vi "OpenSERIAL.vi"(8 "error in (no error)":errorcluster, 9 "Update Rate (4Hz-100Hz)":u8=100, 10 "Protocol":T1=enum."AHRS", 11 "Serial Port":T2=enum."MXP TTL") -> (0 "error out":errorcluster, 3 "navX out":refnum<class "navX.lvclass">)   [LabVIEW 2015, in "navX Library v3.lvlib" / "navX.lvclass"]
uses:
  navX.lvclass
  _NI WPI Serial USB/WPI_SerialPort_USB.ctl
  navX - SERIAL/Protocol.ctl
  navX - SERIAL/navX - SERIAL.lvclass
  navX - SERIAL/navX - SERIAL.lvclass/navX - SERIAL.ctl
  navX - Interface/Notifications/Send Notification.vi
  _NI WPI Serial USB/_NI WPI Serial USB.lvlib
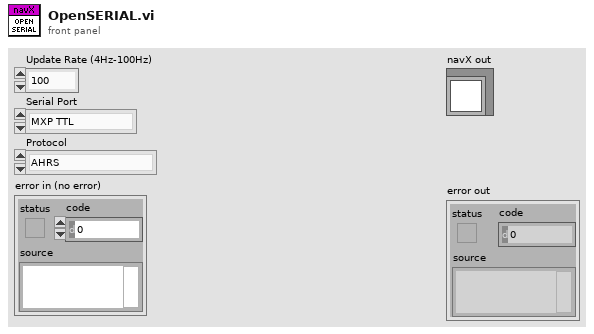
[diagram p1: front panel]
types:
  T1 = typedef "navX Library v3.lvlib/navX - SERIAL.lvclass/Protocol.ctl" = enum16{"YRPH", "Quaterinons", "Gyro/Raw", "AHRS", "AHRSAndPositioning"}
  T2 = typedef "_NI WPI Serial USB.lvlib/WPI_SerialPort_USB.ctl" = enum16{"Onboard RS-232", "MXP TTL", "USB"}
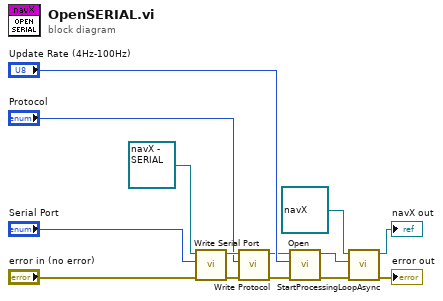
[diagram p0: block diagram]
diagram:
  n1 = call "Write Serial Port.vi"("error in (no error)"="error in (no error)", "Serial Port"="Serial Port", "navX - SERIAL in"=refnum<class "navX - SERIAL.lvclass"> refnum ("navX Library v3.lvlib:navX - SERIAL.lvclass")) -> ("error out"=w11:errorcluster, "navX - SERIAL out"=w12:refnum<class "navX - SERIAL.lvclass">)  [unwired: 7 in]
  n2 = call "Write Protocol.vi"("error in (no error)"=w11, "Protocol"="Protocol", "navX - SERIAL in"=w12) -> ("error out"=w8:errorcluster, "navX - SERIAL out"=w9:refnum<class "navX - SERIAL.lvclass">)  [unwired: 7 in]
  n3 = call-dynamic "Open.vi"("error in (no error)"=w8, "Update Rate (4Hz-100Hz)"="Update Rate (4Hz-100Hz)", "navX - SERIAL in"=w9) -> ("error out"=w5:errorcluster, "navX - SERIAL out"=w4:refnum<class "navX - SERIAL.lvclass">)  [unwired: 7 in]
  n4 = call "StartProcessingLoopAsync.vi"("error in (no error)"=w5, "navX Class in"=w4, "navX in"=refnum<class "navX.lvclass"> refnum ("navX Library v3.lvlib:navX.lvclass")) -> ("error out"=→"error out":errorcluster, "navX out"=→"navX out":refnum<class "navX.lvclass">)  [unwired: 7 in]
